vi "sin.vi"() -> ()   [LabVIEW 2017]
panel:
  out "布尔":bool
  out "数值":dbl
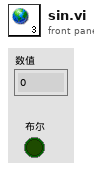
[diagram p1: front panel]
diagram:
